vi "_FPGA_U32equal3.vi"(10 "Numeric":u32) -> (2 "==3?":bool)   [LabVIEW 2018]
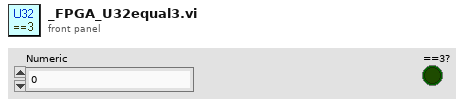
[diagram p1: front panel]
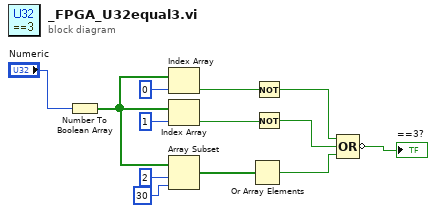
[diagram p0: block diagram]
diagram:
  n1 = Number To Boolean Array(number="Numeric") -> (Boolean array=w4:bool[])
  n2 = Index Array(array=w4, index=0) -> (element=w2:bool)
  n3 = Index Array(array=w4, index=1) -> (element=w9:bool)
  n4 = Array Subset(array=w4, index=2, length=30) -> (w8:bool[])
  n5 = Or Array Elements(Boolean array=w8) -> (logical OR=w6:bool)
  n6 = Not(x=w2) -> (.not. x?=w1:bool)
  n7 = Not(x=w9) -> (.not. x?=w7:bool)
  n8 = Compound Arithmetic op=OR(w1, w7, w6) -> (invert →"==3?":bool)
